vi "Test Generated Mock Class Overrides Dynamic Dispatch VI.vi"(8 "error in (no error)":errorcluster, 11 "Test Case In":refnum<class "Pure Mock Class Generator Test.lvclass">) -> (0 "error out":errorcluster, 3 "Test Case Out":refnum<class "Pure Mock Class Generator Test.lvclass">)   [LabVIEW 2020, in "Pure Mock Class Generator Test.lvclass"]
uses:
  Pure Mock Class Generator Test.lvclass
  C:/Program Files (x86)/National Instruments/LabVIEW 2020/vi.lib/Astemes/LUnit/Test Case.lvclass
  <vilib>/Astemes/LUnit/Test Case.lvclass/Test Case.ctl
  d61b9b24-4b0f-44ef-a9bb-4996cb077d5f.vi
  <vilib>/Astemes/LUnit/Append Pass Result.vi
  <vilib>/Astemes/LUnit/Append Fail Result.vi
  <vilib>/Astemes/LUnit/Describe Comparison.vi
  <vilib>/Astemes/LUnit/Compare Variants.vi
  <vilib>/Astemes/LUnit/Variant to string.vi
  <vilib>/Utility/Data Type/Get Type Information.vi
  <vilib>/Utility/LVClass/Get LV Class Name.vi
  source/Scripting/Interface Identifier/Interface Identifier.lvclass
  source/Scripting/Pure Mock Class Generator/Pure Mock Class Generator.lvclass
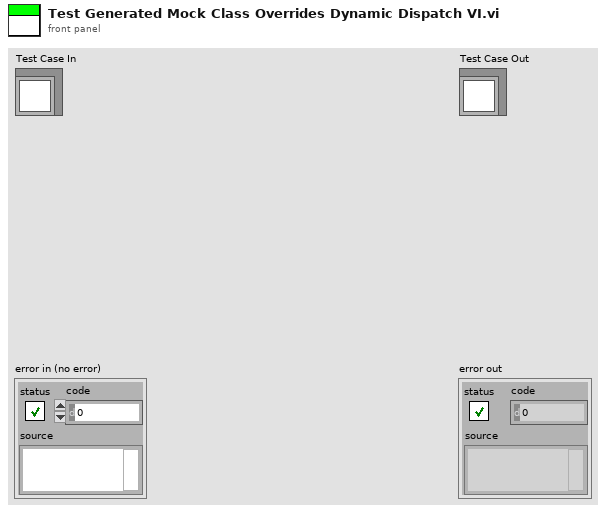
[diagram p1: front panel]
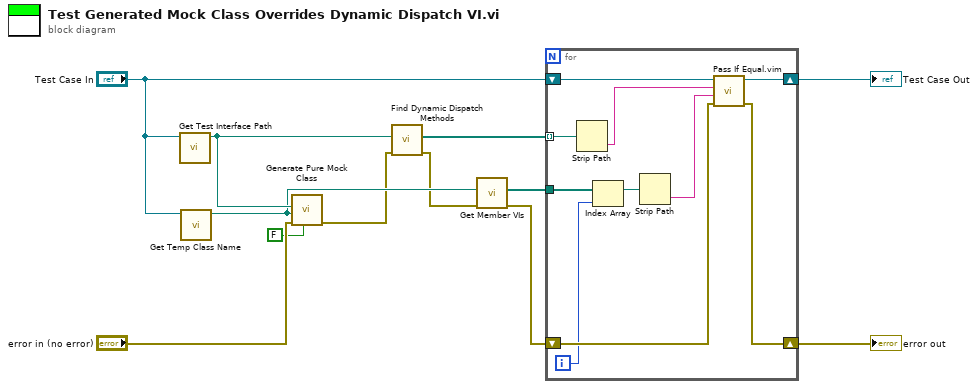
[diagram p0: block diagram]
diagram:
  n1 = call "Get Test Interface Path.vi"("Mock Class Generator Test in"="Test Case In") -> ("Test Class Path"=w8:path)  [unwired: 10 in]
  n2 = call "Get Temp Class Name.vi"("Mock Class Generator Test in"="Test Case In") -> ("Test Class Path"=w7:path)  [unwired: 10 in]
  n3 = call "Generate Pure Mock Class.vi"("Add to lvproj?"=FALSE, "error in (no error)"="error in (no error)", "Destination Class Path"=w7, "Source Class Path"=w8) -> ("error out"=w5:errorcluster)  [unwired: 7 in]
  n4 = call "Find Dynamic Dispatch Methods.vi"("error in (no error)"=w5, "Class Path"=w8) -> ("error out"=w6:errorcluster, "Dynamic Dispatch VIs"=w2:path[])  [unwired: 8 in]
  n5 = call "Get Member VIs.vi"("error in (no error)"=w6, "Test Class Path"=w7) -> ("error out"=w4:errorcluster, "Array"=w3:path[])  [unwired: 8 in]
  n6 = for {
    shift-right: [w22] -> w12
    shift-left: "Test Case In" -> [w20]
    shift-right: [w21] -> w11
    shift-left: w4 -> [w19]
    tunnel: w3 -> [w18]
    tunnel: w2 -> [w17] mode=indexing
    i -> [w15]
    n7 = Strip Path(path=w17) -> (name=w14:string)  [unwired: 1 out]
    n8 = Index Array(array=w18, index=w15) -> (element=w16:path)
    n9 = Strip Path(path=w16) -> (name=w13:string)  [unwired: 1 out]
    n10 = call "Pass If Equal.vim"("error in (no error)"=w19, "Actual"=w13, "Expected"=w14, "LUnit Test Case In"=w20) -> ("error out"=w21:errorcluster, "LUnit Test Case Out"=w22:refnum<class "Pure Mock Class Generator Test.lvclass">)  [unwired: 6 in]
  }
  "error out" <- w11
  "Test Case Out" <- w12
